vi "Rinse 2.vi"() -> ()   [LabVIEW 2019]
uses:
  <vilib>/NI/Current Value Table/Type Defs/Single Tag.ctl
  <vilib>/NI/Current Value Table/Type Defs/Data Types.ctl
  <vilib>/Utility/miscctls.llb/LVDateTimeRec.ctl
  <vilib>/NI/STM/TCP/Read Meta Data (TCP Ref).vi
  <vilib>/NI/STM/TCP/Get Connection Reference (TCP).vi
  <vilib>/NI/AMC/Read Termination Message.vi
  <vilib>/NI/AMC/Create Single Message.vi
  <vilib>/NI/AMC/Update Message Routing Info.vi
  <vilib>/NI/STM/TCP/Read Meta Data (TCP Clst).vi
  <vilib>/NI/AMC/Globals.vi
  <vilib>/NI/STM/TCP/Write Message (TCP).vi
  <vilib>/NI/AMC/Send Message.vi
  <vilib>/NI/AMC/AMC.lvlib
  <vilib>/NI/STM/NI STM.lvlib
  <vilib>/NI/Current Value Table/Current Value Table.lvlib
panel:
  out "Valve Position":dbl(knob) scale=0.0..100.0
  out "Since":timestamp
  out "E Stop":bool
  out "Run Enabled?":bool
  in  "Override Rinse (Turn On)":bool
  out "Rinse Water Temperature":dbl(slide) scale=0.0..40.0
  in  "Outgoing Conductivity":dbl(slide) scale=0.1..1000.0
  out "Accumulater Water Usage":dbl
  in  "Valve Setpoint (%)":dbl(knob) min=0.0 max=75.0 step=1.0 scale=10.0..100.0
  in  "Enable Auto Rinse":bool
  out "DI Flow rate":dbl(knob) scale=0.0..80.0
  in  "Machine":bool
  in  "Basement 4":bool
  in  "Dryer":bool
  in  "Rinse 4":bool
  in  "Rinse 3":bool
  in  "Rinse 2":bool
  in  "Basement 3":bool
  in  "Basement 2":bool
  in  "Basement 1":bool
  in  "Plater 6":bool
  in  "Plater 5":bool
  in  "Plater 4":bool
  in  "Plater 3":bool
  in  "Plater 2":bool
  in  "Plater 1":bool
  in  "Predip":bool
  in  "Rinse 1":bool
  in  "Cleaner":bool
  in  "Etch":bool
  out "status":string
  # "Module Selection"
  # "L/min"
  # "µS"
  # "Liters"
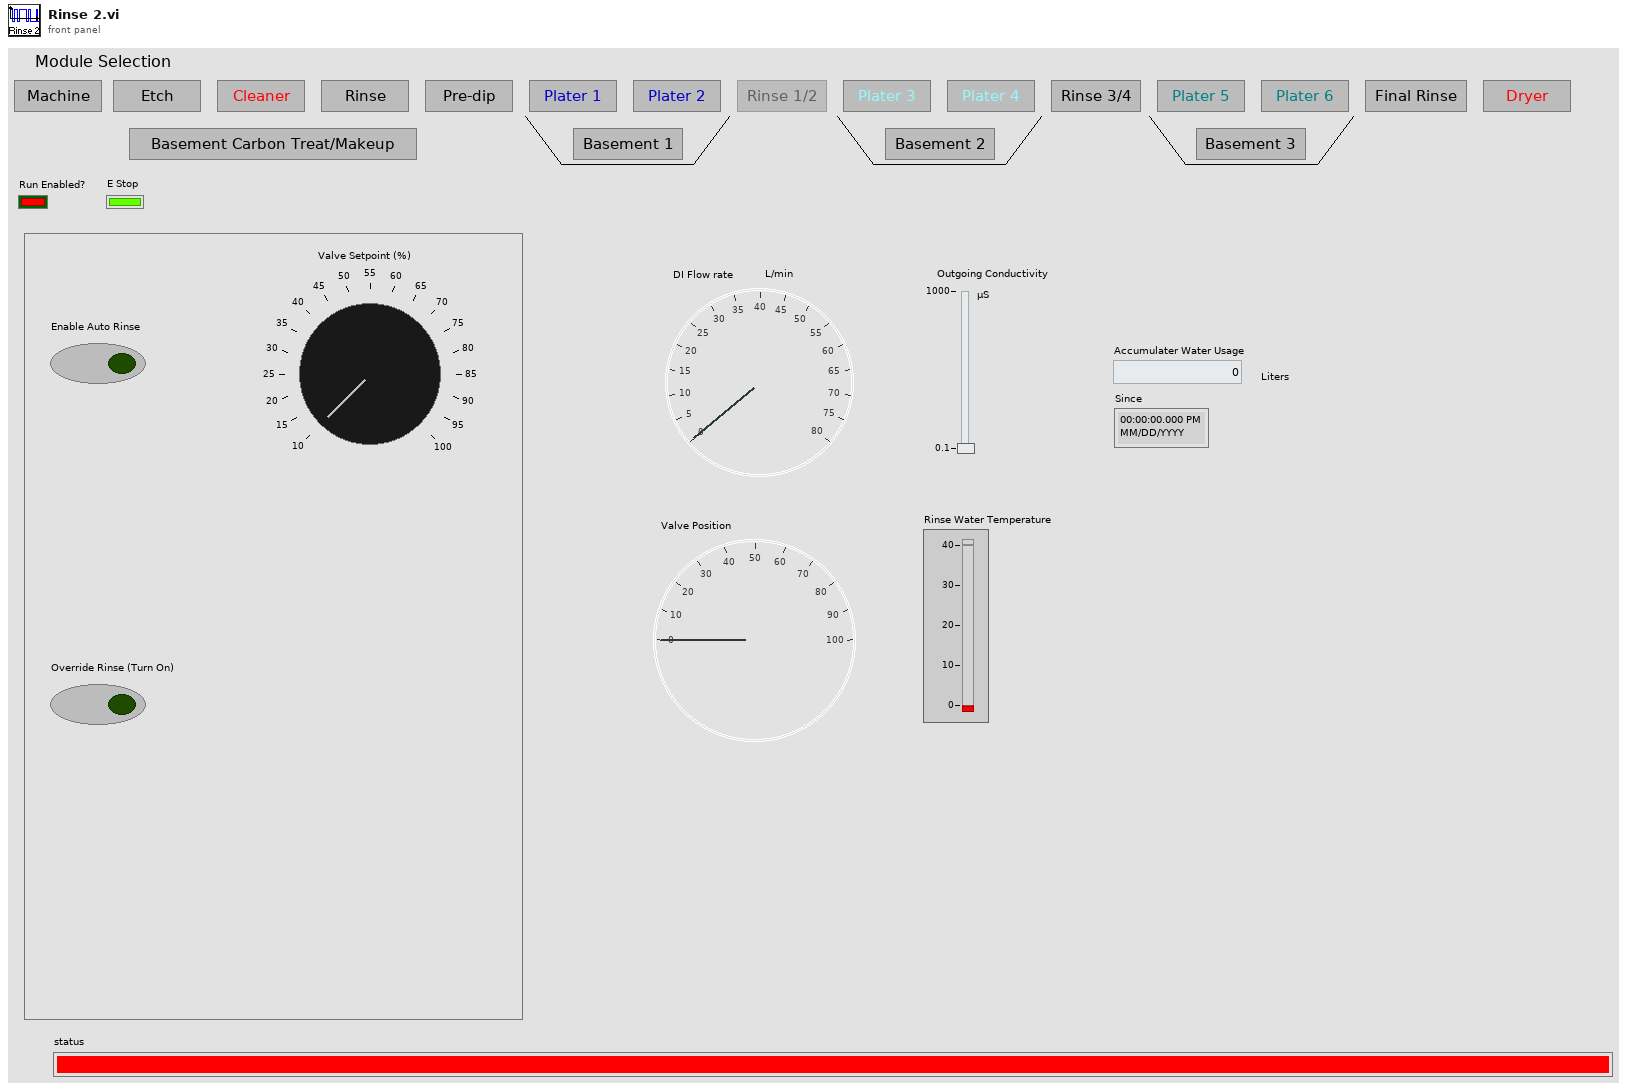
[diagram p1: front panel]
types:
  T1 = typedef "Current Value Table.lvlib/Single Tag.ctl" = cluster{"Data Type":T2, "Name":string, "Value":string, "Description":string}
  T2 = typedef "Current Value Table.lvlib/Data Types.ctl" = enum16{"Double", "Single", "I64", "I32", "I16", "I8", "U64", "U32", "U16", "U8", "String", "Boolean", "Array of U8", "Array of U16", "Array of U32", "Array of U64", "Array of I64", "Array of I32", "Array of I16", "Array of I8", "Array of Double", "Array of Single", "Array of Boolean", "Array of String"}
  T3 = typedef "NI STM.lvlib/TCP Connection Info.ctl" = cluster{"connection ID":refnum<k5>, "meta data":T4[]}
  T4 = typedef "NI STM.lvlib/MetaDataElement.ctl" = string
  T5 = typedef "AMC.lvlib/Message Queue.ctl" = refnum<queue>
  T6 = typedef "LVDateTimeRec.ctl" = cluster{"fractional second":dbl, "second":i32, "minute":i32, "hour":i32, "day of month":i32, "month":i32, "year":i32, "day of week":i32, "day of year":i32, "DST":i32}
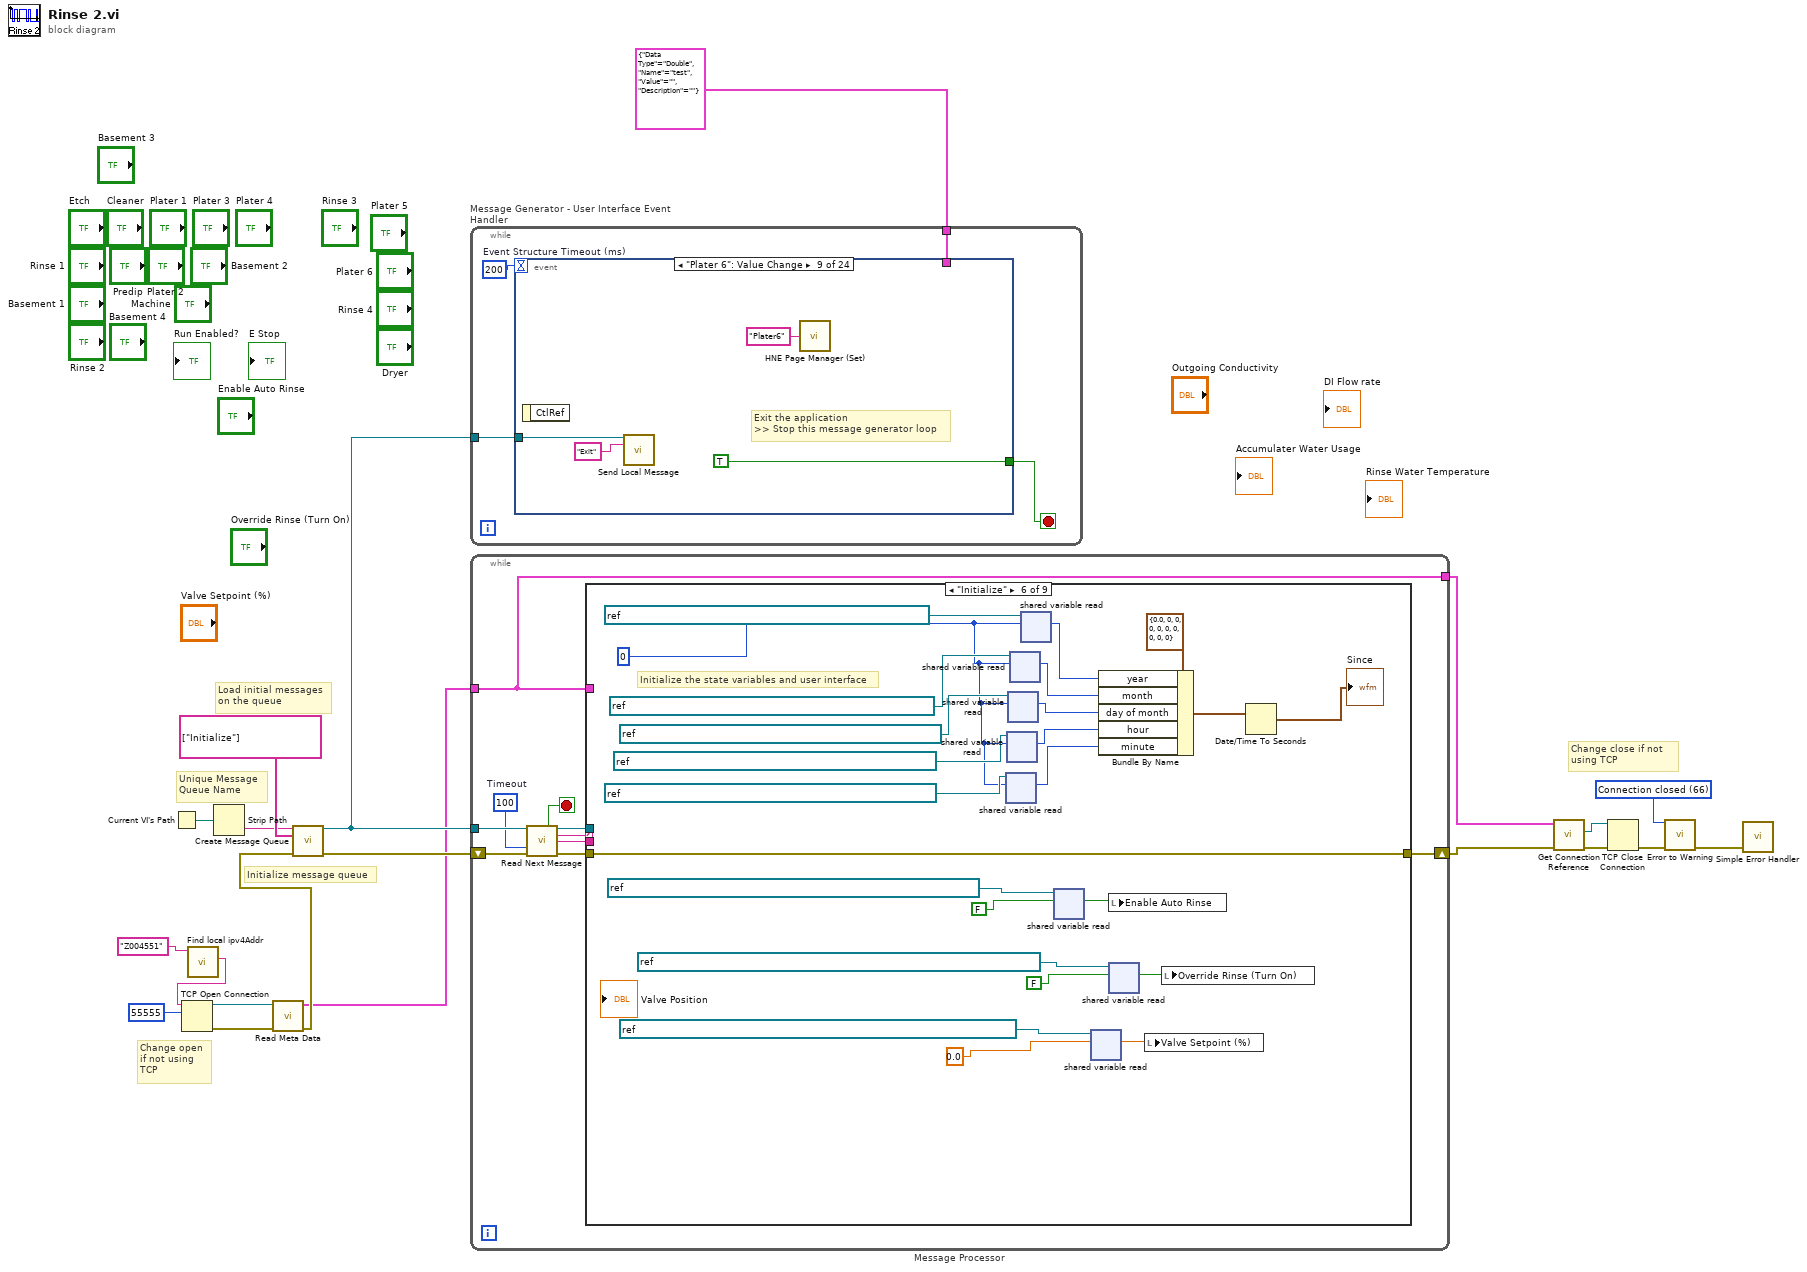
[diagram p0: block diagram]
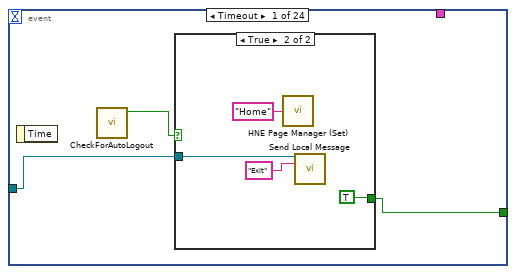
[diagram p2: hidden frame]
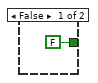
[diagram p3: hidden frame]
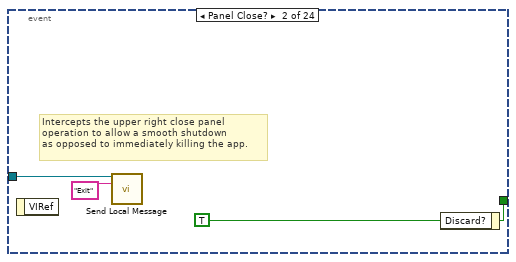
[diagram p4: hidden frame]
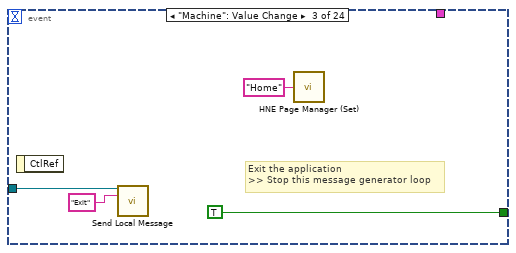
[diagram p5: hidden frame]
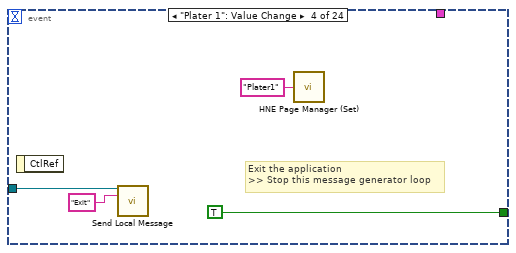
[diagram p6: hidden frame]
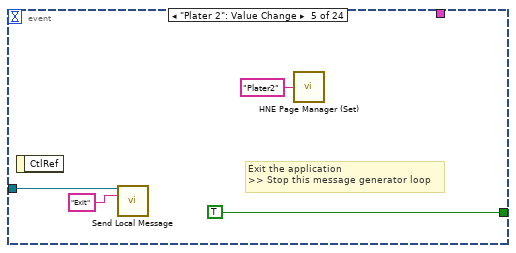
[diagram p7: hidden frame]
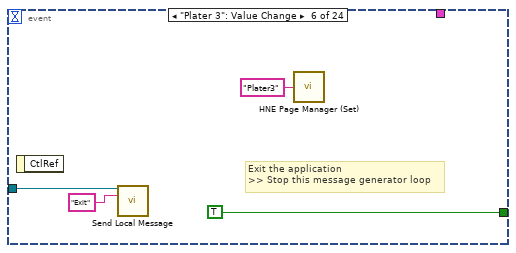
[diagram p8: hidden frame]
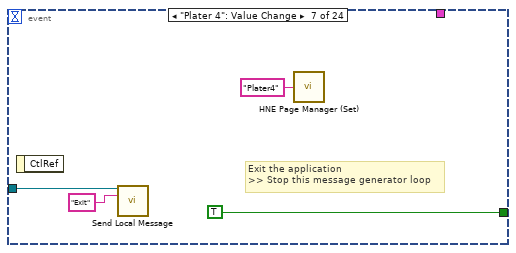
[diagram p9: hidden frame]
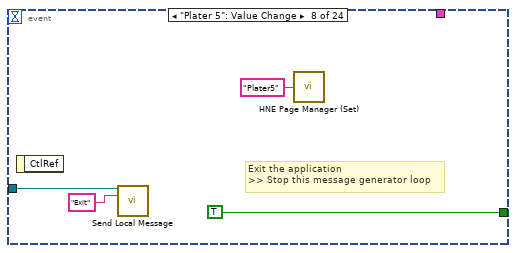
[diagram p10: hidden frame]
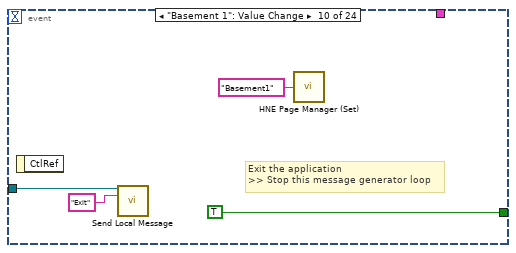
[diagram p11: hidden frame]
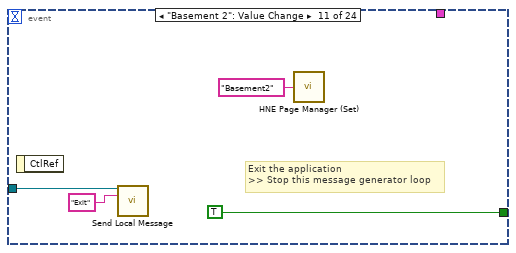
[diagram p12: hidden frame]
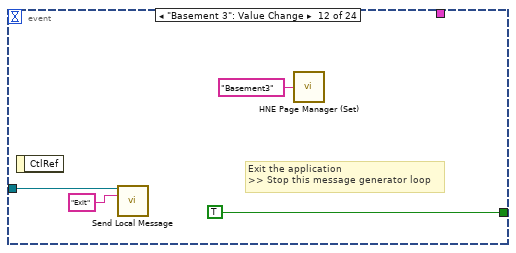
[diagram p13: hidden frame]
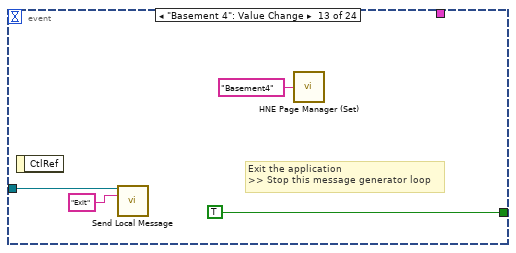
[diagram p14: hidden frame]
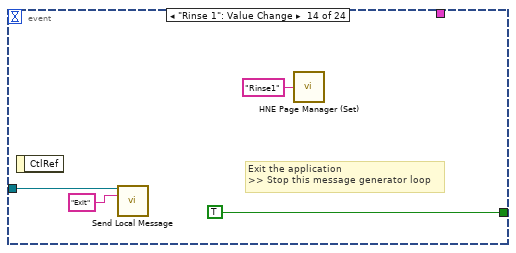
[diagram p15: hidden frame]
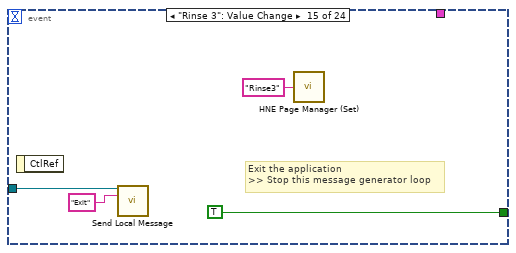
[diagram p16: hidden frame]
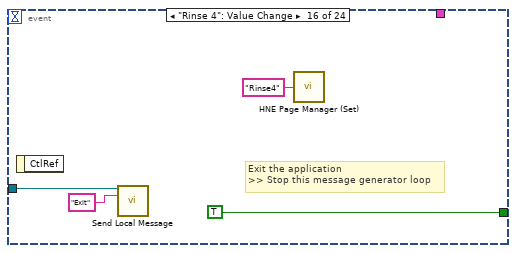
[diagram p17: hidden frame]
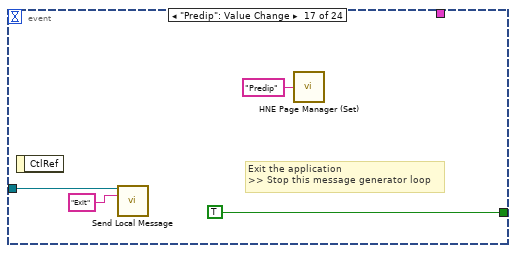
[diagram p18: hidden frame]
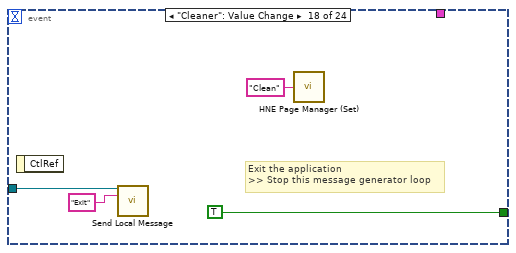
[diagram p19: hidden frame]
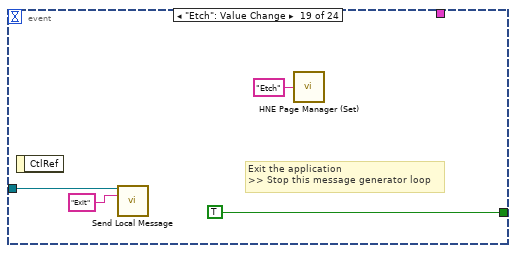
[diagram p20: hidden frame]
diagram:
  w9 = 66 items=["No Error", "Argument Error", "Memory Full", "Out of Zone", "End of File", "File Already Open", "Generic File IO Error", "File Not Found", "File Permission Error", "Disk Full", "Duplicate Path", "Too Many Files Open", "Not Enabled", "Resource File Not Found", "Cannot Add Resource", "Resource Not Found", "Image Not Found", "Image Memory Error", "Pen Does Not Exist", "Config Bad Type", "Config Token Not Found", "Config Parse Error", "Config Memory Error", "Bad External Code Format", "Bad External Code Offset", "External Code Not Present", "Null Window", "Destroy Window Mixup", "Null Menu", "Print Aborted", "Bad Print Record", "Print Driver Error", "Windows Error During Print", "Memory Error During Print", "Print Dialog Error", "Generic Print Error", "Invalid Device Refnum", "Device Not Found", "Device Parameter Error", "Device Unit Error", "Can't Open Device", "Device Call Aborted", "Generic Error", "Cancelled By User", "Object ID Too Low", "Object ID Too High", "Object Not In Heap", "Unknown Heap", "Bad DefProc ID", "DefProc Not In Table", "Message Out Of Range", "Null Method", "Unknown Message", "Manager Call Not Supported", "Bad address", "Connection In progress", "Connection timed out", "Connection is already in progress", "Network attribute not supported", "Network error", "Address in use", "System out of memory", "Connection aborted", "Connection refused", "Connection is not connected", "Connection is already connected", "Connection closed", "Initialize error (interapplication manager)", "Bad occurrence", "Wait on unbound occurrence handler", "Occurrence queue overflow", "Bad path", "Semaphore not signaled", "Unrecognized type (interapplication manager)"] ("1st Error to Convert")
  # "Change close if not using TCP"
  # "Change open if not using TCP"
  # "Initialize message queue"
  # "Unique Message\nQueue Name"
  # "Load initial messages\non the queue"
  n1 = Current VI's Path() -> (path=w16:path)
  n2 = call "Find local ipv4Addr.vi"("MachineToFind"="Z004551" ("Target IP Address")) -> ("name"=w2:string)  [unwired: 9 in, 1 out]
  n3 = TCP Open Connection(address=w2, remote port or service name=u16 55555 ("remote port")) -> (connection ID=w14:refnum<k5>, error out=w13:errorcluster)  [unwired: 1 in, 2 out]
  n4 = Strip Path(path=w16) -> (name=w19:string)  [unwired: 1 out]
  n5 = call-poly <vilib>:"Read Meta Data.vi"("error in"=w13, "connection ID"=w14) -> ("error out"=w12:errorcluster, "connection info out"=w11:T3)  [unwired: 7 in, 1 out]
  n6 = call <vilib>:"Create Message Queue.vi"("message queue name"=w19, "initial message names"=string[] ["Initialize"], "error in"=w12) -> ("message queue out"=w18:T5, "error out"=w17:errorcluster)  [unwired: 11 in]
  n7 = while "Message Generator - User Interface Event Handler" {
    tunnel: w18 -> [w22]
    tunnel: T1 {"Data Type"=enum."Double", "Name"="test", "Value"="", "Description"=""} ("Tag") -> [w21]
    stop <- w23 stop-if-true
    w24 = 200  # Event Structure Timeout (ms)
    n8 = event shown="[8] \"Plater 6\": Value Change" {
      selector: _ -> [_ _ _ _ _ _ _ _ _ _ _ _ _ _ _ _ _ _ _ _ _ _ _ _]
      dyn-events: _ -> [_ _ _ _ _ _ _ _ _ _ _ _ _ _ _ _ _ _ _ _ _ _ _ _]
      timeout: w24 -> [_ _ _ _ _ _ _ _ _ _ _ _ _ _ _ _ _ _ _ _ _ _ _ _]
      tunnel: [w25 w35 TRUE ("Discard?") TRUE ("Discard?") TRUE ("Discard?") TRUE ("Discard?") TRUE ("Discard?") TRUE ("Discard?") TRUE ("Discard?") TRUE ("Discard?") TRUE ("Discard?") TRUE ("Discard?") TRUE ("Discard?") TRUE ("Discard?") TRUE ("Discard?") TRUE ("Discard?") TRUE ("Discard?") TRUE ("Discard?") TRUE ("Discard?") TRUE ("Discard?") FALSE ("Discard?") FALSE ("Discard?") FALSE ("Discard?") _] -> w23
      tunnel: w22 -> [w26 w33 w37 w41 w45 w49 w53 w57 w61 w65 w69 w73 w77 w81 w85 w89 w93 w97 w101 w105 w116 w127 w137 w140]
      tunnel: w21 -> [_ _ _ _ _ _ _ _ _ _ _ _ _ _ _ _ _ _ _ _ w110 w121 w133 _]
      event Timeout {
        n9 = event-data() -> ()  [unwired: 2 out]
        n10 = call "CheckForAutoLogout.vi"() -> ("Boolean"=w27:bool)  [unwired: 11 in]
        n11 = case shown="True" w27 {
          tunnel: [FALSE ("Discard?") TRUE ("Discard?")] -> w25
          tunnel: w26 -> [_ w29]
          frame False {
          }
          frame True {
            n12 = call <userlib>:"HNE Page Manager (Set).vi"("Next Page"="Home") -> ()  [unwired: 4 in, 1 out]
            n13 = call <vilib>:"Send Local Message.vi"("message queue in"=w29, "message name"="Exit") -> ()  [unwired: 11 in, 3 out]
          }
        }
      }
      event Panel Close? {
        w35 = TRUE ("Discard?")
        # "Intercepts the upper right close panel\noperation to allow a smooth shutdown\nas opposed to immediately killing the app."
        n14 = event-data() -> ()  [unwired: 2 out]
        n15 = call <vilib>:"Send Local Message.vi"("message queue in"=w33, "message name"="Exit") -> ()  [unwired: 11 in, 3 out]
        n16 = event-data("Discard?"=w35) -> ()  [unwired: 1 in, 1 out]
      }
      event "Machine": Value Change {
        # "Exit the application\n>> Stop this message generator loop"
        n17 = event-data() -> ()  [unwired: 2 out]
        n18 = call <vilib>:"Send Local Message.vi"("message queue in"=w37, "message name"="Exit") -> ()  [unwired: 11 in, 3 out]
        n19 = call <userlib>:"HNE Page Manager (Set).vi"("Next Page"="Home") -> ()  [unwired: 4 in, 1 out]
      }
      event "Plater 1": Value Change {
        # "Exit the application\n>> Stop this message generator loop"
        n20 = event-data() -> ()  [unwired: 2 out]
        n21 = call <vilib>:"Send Local Message.vi"("message queue in"=w41, "message name"="Exit") -> ()  [unwired: 11 in, 3 out]
        n22 = call <userlib>:"HNE Page Manager (Set).vi"("Next Page"="Plater1") -> ()  [unwired: 4 in, 1 out]
      }
      event "Plater 2": Value Change {
        # "Exit the application\n>> Stop this message generator loop"
        n23 = event-data() -> ()  [unwired: 2 out]
        n24 = call <vilib>:"Send Local Message.vi"("message queue in"=w45, "message name"="Exit") -> ()  [unwired: 11 in, 3 out]
        n25 = call <userlib>:"HNE Page Manager (Set).vi"("Next Page"="Plater2") -> ()  [unwired: 4 in, 1 out]
      }
      event "Plater 3": Value Change {
        # "Exit the application\n>> Stop this message generator loop"
        n26 = event-data() -> ()  [unwired: 2 out]
        n27 = call <vilib>:"Send Local Message.vi"("message queue in"=w49, "message name"="Exit") -> ()  [unwired: 11 in, 3 out]
        n28 = call <userlib>:"HNE Page Manager (Set).vi"("Next Page"="Plater3") -> ()  [unwired: 4 in, 1 out]
      }
      event "Plater 4": Value Change {
        # "Exit the application\n>> Stop this message generator loop"
        n29 = event-data() -> ()  [unwired: 2 out]
        n30 = call <vilib>:"Send Local Message.vi"("message queue in"=w53, "message name"="Exit") -> ()  [unwired: 11 in, 3 out]
        n31 = call <userlib>:"HNE Page Manager (Set).vi"("Next Page"="Plater4") -> ()  [unwired: 4 in, 1 out]
      }
      event "Plater 5": Value Change {
        # "Exit the application\n>> Stop this message generator loop"
        n32 = event-data() -> ()  [unwired: 2 out]
        n33 = call <vilib>:"Send Local Message.vi"("message queue in"=w57, "message name"="Exit") -> ()  [unwired: 11 in, 3 out]
        n34 = call <userlib>:"HNE Page Manager (Set).vi"("Next Page"="Plater5") -> ()  [unwired: 4 in, 1 out]
      }
      event "Plater 6": Value Change {
        # "Exit the application\n>> Stop this message generator loop"
        n35 = event-data() -> ()  [unwired: 2 out]
        n36 = call <vilib>:"Send Local Message.vi"("message queue in"=w61, "message name"="Exit") -> ()  [unwired: 11 in, 3 out]
        n37 = call <userlib>:"HNE Page Manager (Set).vi"("Next Page"="Plater6") -> ()  [unwired: 4 in, 1 out]
      }
      event "Basement 1": Value Change {
        # "Exit the application\n>> Stop this message generator loop"
        n38 = event-data() -> ()  [unwired: 2 out]
        n39 = call <vilib>:"Send Local Message.vi"("message queue in"=w65, "message name"="Exit") -> ()  [unwired: 11 in, 3 out]
        n40 = call <userlib>:"HNE Page Manager (Set).vi"("Next Page"="Basement1") -> ()  [unwired: 4 in, 1 out]
      }
      event "Basement 2": Value Change {
        # "Exit the application\n>> Stop this message generator loop"
        n41 = event-data() -> ()  [unwired: 2 out]
        n42 = call <vilib>:"Send Local Message.vi"("message queue in"=w69, "message name"="Exit") -> ()  [unwired: 11 in, 3 out]
        n43 = call <userlib>:"HNE Page Manager (Set).vi"("Next Page"="Basement2") -> ()  [unwired: 4 in, 1 out]
      }
      event "Basement 3": Value Change {
        # "Exit the application\n>> Stop this message generator loop"
        n44 = event-data() -> ()  [unwired: 2 out]
        n45 = call <vilib>:"Send Local Message.vi"("message queue in"=w73, "message name"="Exit") -> ()  [unwired: 11 in, 3 out]
        n46 = call <userlib>:"HNE Page Manager (Set).vi"("Next Page"="Basement3") -> ()  [unwired: 4 in, 1 out]
      }
      event "Basement 4": Value Change {
        # "Exit the application\n>> Stop this message generator loop"
        n47 = event-data() -> ()  [unwired: 2 out]
        n48 = call <vilib>:"Send Local Message.vi"("message queue in"=w77, "message name"="Exit") -> ()  [unwired: 11 in, 3 out]
        n49 = call <userlib>:"HNE Page Manager (Set).vi"("Next Page"="Basement4") -> ()  [unwired: 4 in, 1 out]
      }
      event "Rinse 1": Value Change {
        # "Exit the application\n>> Stop this message generator loop"
        n50 = event-data() -> ()  [unwired: 2 out]
        n51 = call <vilib>:"Send Local Message.vi"("message queue in"=w81, "message name"="Exit") -> ()  [unwired: 11 in, 3 out]
        n52 = call <userlib>:"HNE Page Manager (Set).vi"("Next Page"="Rinse1") -> ()  [unwired: 4 in, 1 out]
      }
      event "Rinse 3": Value Change {
        # "Exit the application\n>> Stop this message generator loop"
        n53 = event-data() -> ()  [unwired: 2 out]
        n54 = call <vilib>:"Send Local Message.vi"("message queue in"=w85, "message name"="Exit") -> ()  [unwired: 11 in, 3 out]
        n55 = call <userlib>:"HNE Page Manager (Set).vi"("Next Page"="Rinse3") -> ()  [unwired: 4 in, 1 out]
      }
      event "Rinse 4": Value Change {
        # "Exit the application\n>> Stop this message generator loop"
        n56 = event-data() -> ()  [unwired: 2 out]
        n57 = call <vilib>:"Send Local Message.vi"("message queue in"=w89, "message name"="Exit") -> ()  [unwired: 11 in, 3 out]
        n58 = call <userlib>:"HNE Page Manager (Set).vi"("Next Page"="Rinse4") -> ()  [unwired: 4 in, 1 out]
      }
      event "Predip": Value Change {
        # "Exit the application\n>> Stop this message generator loop"
        n59 = event-data() -> ()  [unwired: 2 out]
        n60 = call <vilib>:"Send Local Message.vi"("message queue in"=w93, "message name"="Exit") -> ()  [unwired: 11 in, 3 out]
        n61 = call <userlib>:"HNE Page Manager (Set).vi"("Next Page"="Predip") -> ()  [unwired: 4 in, 1 out]
      }
      event "Cleaner": Value Change {
        # "Exit the application\n>> Stop this message generator loop"
        n62 = event-data() -> ()  [unwired: 2 out]
        n63 = call <vilib>:"Send Local Message.vi"("message queue in"=w97, "message name"="Exit") -> ()  [unwired: 11 in, 3 out]
        n64 = call <userlib>:"HNE Page Manager (Set).vi"("Next Page"="Clean") -> ()  [unwired: 4 in, 1 out]
      }
      event "Etch": Value Change {
        # "Exit the application\n>> Stop this message generator loop"
        n65 = event-data() -> ()  [unwired: 2 out]
        n66 = call <vilib>:"Send Local Message.vi"("message queue in"=w101, "message name"="Exit") -> ()  [unwired: 11 in, 3 out]
        n67 = call <userlib>:"HNE Page Manager (Set).vi"("Next Page"="Etch") -> ()  [unwired: 4 in, 1 out]
      }
      event "Dryer": Value Change {
        # "Exit the application\n>> Stop this message generator loop"
        n68 = event-data() -> ()  [unwired: 2 out]
        n69 = call <vilib>:"Send Local Message.vi"("message queue in"=w105, "message name"="Exit") -> ()  [unwired: 11 in, 3 out]
        n70 = call <userlib>:"HNE Page Manager (Set).vi"("Next Page"="Dryer") -> ()  [unwired: 4 in, 1 out]
      }
      event "Enable Auto Rinse": Value Change {
        n71 = event-data() -> ("NewVal"=w115:bool)  [unwired: 6 out]
        n72 = Boolean To (0,1)(Boolean=w115) -> (0, 1=w114:i16)
        n73 = Number To Decimal String(number=w114) -> (decimal integer string=w109:string)  [unwired: 1 in]
        n74 = Bundle By Name(cluster=w110, "Data Type"=Data_Types."Boolean", "Name"="HMI_Enable_Rinse2", "Value"=w109) -> (w111:T1)
        n75 = Flatten To String(anything=w111) -> (data string=w108:string)  [unwired: 3 in, 2 out]
        n76 = call <vilib>:"Send Local Message.vi"("message queue in"=w116, "message name"="Write_Tag", "message value"=w108) -> ()  [unwired: 10 in, 3 out]
      }
      event "Override Rinse (Turn On)": Value Change {
        n77 = event-data() -> ("NewVal"=w126:bool)  [unwired: 6 out]
        n78 = Boolean To (0,1)(Boolean=w126) -> (0, 1=w125:i16)
        n79 = Number To Decimal String(number=w125) -> (decimal integer string=w120:string)  [unwired: 1 in]
        n80 = Bundle By Name(cluster=w121, "Data Type"=Data_Types."Boolean", "Name"="HMI_Rinse2_OverrideRun", "Value"=w120) -> (w122:T1)
        n81 = Flatten To String(anything=w122) -> (data string=w119:string)  [unwired: 3 in, 2 out]
        n82 = call <vilib>:"Send Local Message.vi"("message queue in"=w127, "message name"="Write_Tag", "message value"=w119) -> ()  [unwired: 10 in, 3 out]
      }
      event "Valve Setpoint (%)": Value Change {
        n83 = event-data() -> ("NewVal"=w131:dbl)  [unwired: 6 out]
        n84 = Number To Fractional String(number=w131) -> (F-format string=w130:string)  [unwired: 3 in]
        n85 = Bundle By Name(cluster=w133, "Data Type"=Data_Types."Double", "Name"="HMI_Rinse2_VlvSetpoint", "Value"=w130) -> (w134:T1)
        n86 = Flatten To String(anything=w134) -> (data string=w132:string)  [unwired: 3 in, 2 out]
        n87 = call <vilib>:"Send Local Message.vi"("message queue in"=w137, "message name"="Write_Tag", "message value"=w132) -> ()  [unwired: 10 in, 3 out]
      }
      event Menu Selection (User) {
        # "Add run-time menu items to the message\nqueue. The message handler case names must match the menu ItemTag names."
        n88 = event-data() -> ("ItemTag"=w141:string)  [unwired: 1 out]
        n89 = call <vilib>:"Send Local Message.vi"("message queue in"=w140, "message name"=w141) -> ()  [unwired: 11 in, 3 out]
      }
    }
  }
  n90 = while "Message Processor" {
    shift-left: w17 -> [w147]
    shift-right: [w151] -> w4
    tunnel: w18 -> [w148]
    tunnel: w11 -> [w142]
    tunnel: [w142] -> w5
    stop <- w150 stop-if-true
    w143 = 100  # Timeout
    n91 = call <vilib>:"Read Next Message.vi"("message queue in"=w148, "timeout (1 ms)"=w143, "error in"=w147) -> ("exit process?"=w150:bool, "message queue out"=w149:T5, "message name"=w145:string, "message value"=w144:string, "error out"=w146:errorcluster)  [unwired: 5 in, 3 out]
    n92 = case shown="\"Initialize\"" w145 {
      selector: w145 -> [_ _ w162 _ _ _ _ _ _]
      tunnel: w149 -> [_ _ _ _ _ _ w192 _ _]
      tunnel: w146 -> [w152 w159 w163 w164 w166 w190 w193 w195 w199]
      tunnel: [w152 w159 w163 errorcluster {"status"=FALSE, "code"=0, "source"=""} ("error out") w166 w190 w191 w195 w198] -> w151
      tunnel: w144 -> [_ _ _ _ _ _ _ _ w196]
      tunnel: w142 -> [_ _ _ _ _ _ _ _ w197]
      frame "---------- Framework Operations ----------" {
        # "Dummy case to add a seperator in the Case Structure menu"
      }
      frame "", "Idle" {
        # "Update the front panel"
        # "Idle Case - this case is called after a Timeout on the Get Next Message from Queue VI, if no new messages are present on the queue. This case can be used for housekeeping tasks such as updating the UI."
        n93 = Get Date/Time String(want seconds? (F)=TRUE) -> (date string=w158:string, time string=w157:string)  [unwired: 2 out]
        n94 = Concatenate Strings(w158, " " ("string"), w157) -> (→"status":string)
        n95 = control-ref of="status"() -> (w153:refnum<vi>)
        n96 = call <userlib>:"TAE Format Alarm Ticker.vi"("Alarm Ticker Ref"=w153) -> ()  [unwired: 15 in]
      }
      frame "Missing Message Handler", Default {
        # "Call this case if a message is received that is not handled \nby any other case. Typically this is a programming error\nas a result of a typo or unhandled message/missing message handler."
        n97 = Format Into String(format string="DevError: Missing message handler for '%s\" message." ("message"), w162) -> (resulting string=w160:string)  [unwired: 2 in, 1 out]
        n98 = One Button Dialog(message=w160) -> ()  [unwired: 2 out]
      }
      frame "Error" {
        # "General Error Case - this case is called if an error is passed using the error cluster below. Typically most new errors should be handed in each individual case and not passed in the rror cluster. If necessary a custom error handler case should be added and called from other cases."
        n99 = call <vilib>:"Simple Error Handler.vi"("error in (no error)"=w164) -> ()  [unwired: 1 in, 8 out]
      }
      frame "---------- Generic Operations ----------" {
        # "Dummy case to add a seperator in the Case Structure menu"
      }
      frame "Initialize" {
        w171 = u32 0
        # "Initialize the state variables and user interface"
        n100 = shared-variable-read(refnum<k21> "ni.var.psp://z004551/CDL0100 ReadTags/Rinse2_Reset_Mn" ("shared variable refnum in"), w171) -> (w170:u32)  [unwired: 1 in, 3 out]
        n101 = shared-variable-read(refnum<k21> "ni.var.psp://z004551/CDL0100 ReadTags/Rinse2_Reset_H" ("shared variable refnum in"), w171) -> (w173:u32)  [unwired: 1 in, 3 out]
        n102 = shared-variable-read(refnum<k21> "ni.var.psp://z004551/CDL0100 ReadTags/Rinse2_Reset_D" ("shared variable refnum in"), w171) -> (w175:u32)  [unwired: 1 in, 3 out]
        n103 = shared-variable-read(refnum<k21> "ni.var.psp://z004551/CDL0100 ReadTags/Rinse2_Reset_M" ("shared variable refnum in"), w171) -> (w177:u32)  [unwired: 1 in, 3 out]
        n104 = shared-variable-read(refnum<k21> "ni.var.psp://z004551/CDL0100 ReadTags/Rinse2_Reset_Yr" ("shared variable refnum in"), w171) -> (w179:u32)  [unwired: 1 in, 3 out]
        n105 = shared-variable-read(refnum<k21> "ni.var.psp://z004551/CDL0100 ReadWriteTags/HMI_Enable_Rinse2" ("shared variable refnum in"), FALSE) -> (w187:bool)  [unwired: 1 in, 3 out]
        n106 = shared-variable-read(refnum<k21> "ni.var.psp://z004551/CDL0100 ReadWriteTags/HMI_Rinse2_VlvSetpoint" ("shared variable refnum in"), 0.0) -> (w167:dbl)  [unwired: 1 in, 3 out]
        n107 = Bundle By Name(cluster=T6 {"fractional second"=0.0, "second"=0, "minute"=0, "hour"=0, "day of month"=0, "month"=0, "year"=0, "day of week"=0, "day of year"=0, "DST"=0} ("date time rec"), "year"=w179, "month"=w177, "day of month"=w175, "hour"=w173, "minute"=w170) -> (w182:T6)
        n108 = local write "Enable Auto Rinse"(w187) -> ()
        n109 = shared-variable-read(refnum<k21> "ni.var.psp://z004551/CDL0100 ReadWriteTags/HMI_Rinse2_OverrideRun" ("shared variable refnum in"), FALSE) -> (w184:bool)  [unwired: 1 in, 3 out]
        n110 = local write "Valve Setpoint (%)"(w167) -> ()
        n111 = local write "Override Rinse (Turn On)"(w184) -> ()
        n112 = Date/Time To Seconds(2:w182) -> (0:→"Since":timestamp)  [unwired: 1 in]
      }
      frame "Exit" {
        # "Destroy message queue >> this will halt the UI event handler loop"
        # "Stop the VI\n>> Perform any cleanup tasks in this message case.\n>> Clear display before closing."
        n113 = call <vilib>:"Destroy Message Queue.vi"("message queue in"=w192, "error in"=w193) -> ("error out"=w191:errorcluster)  [unwired: 11 in, 2 out]
        n114 = local write "status"("" ("Status")) -> ()
      }
      frame "---------- Application Operations ----------" {
        # "Dummy case to add a seperator in the Case Structure menu"
      }
      frame "Write_Tag" {
        n115 = call-poly <vilib>:"Write Message.vi"("error in"=w199, "data"=w196, "name"="WriteTag", "connection info in"=w197) -> ("error out"=w198:errorcluster)  [unwired: 6 in, 1 out]
      }
    }
  }
  n116 = call-poly <vilib>:"Get Connection Reference.vi"("error in"=w4, "connection info in"=w5) -> ("error out"=w8:errorcluster, "connection ID out"=w7:refnum<k5>)  [unwired: 8 out]
  n117 = TCP Close Connection(connection ID=w7, error in (no error)=w8) -> (error out=w10:errorcluster)  [unwired: 2 out]
  n118 = call <vilib>:"Error to Warning.vi"("1st Error to Convert"=w9, "error in"=w10) -> ("warning out"=w6:errorcluster)  [unwired: 3 in, 10 out]
  n119 = call <vilib>:"Simple Error Handler.vi"("error in (no error)"=w6) -> ()  [unwired: 4 in, 5 out]
